vi "_DServerEventHandler.vi"(3 "error in":errorcluster, 4 "dserver evt.":T1, 5 "timeout":i32=250) -> (0 "error out":errorcluster, 1 "client request":T2={"Request Id"=0, "Source Id"=0, "Request Type"=enum."UNKNOWN_REQUEST", "Device Class Name"="unspecified_cmd_or_attr_name", "Device Name"="unspecified/device/name", "Cmd or Attr Name"="unspecified_cmd_or_attr_name", "Client Request Data"={"write attribute value"={"dimx"=0, "dimy"=0, "data"=[], "data_type"=enum."UNKNOWN_DATA_TYPE"}, "exec. command argin"={"num data"=[], "str data"=[]}}}, 2 "timeout":bool)   [LabVIEW 2014, in "tango.lvlib"]
uses:
  tango.lvlib
  Orphan/Typedefs/_DServerClientRequest.ctl
  Orphan/Typedefs/_DServerClientRequestType.ctl
  Orphan/Typedefs/_DServerClientRequestData.ctl
  Orphan/Typedefs/_GenericDataBuffer.ctl
  Orphan/Typedefs/_DataType.ctl
  Orphan/Typedefs/_DServerEvent.ctl
panel:
  in  "client request":T2={"Request Id"=0, "Source Id"=3, "Request Type"=enum."UNKNOWN_REQUEST", "Device Class Name"="unspecified_cmd_or_attr_name", "Device Name"="unspecified/device/name", "Cmd or Attr Name"="unspecified_cmd_or_attr_name", "Client Request Data"={"write attribute value"={"dimx"=0, "dimy"=0, "data"=[], "data_type"=enum."UNKNOWN_DATA_TYPE"}, "exec. command argin"={"num data"=[], "str data"=[]}}}
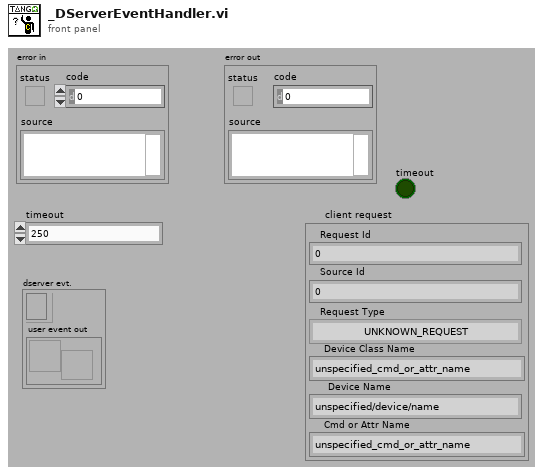
[diagram p1: front panel]
types:
  T1 = typedef "tango.lvlib/_DServerEvent.ctl" = cluster{"event registration refnum":refnum<event-registration>, "user event out":refnum<user-event>}
  T2 = typedef "tango.lvlib/_DServerClientRequest.ctl" = cluster{"Request Id":u32, "Source Id":u32, "Request Type":T3, "Device Class Name":string, "Device Name":string, "Cmd or Attr Name":string, "Client Request Data":T4}
  T3 = typedef "tango.lvlib/_DServerClientRequestType.ctl" = enum16{"EXEC_CMD", "READ_ATTR", "WRITE_ATTR", "UNKNOWN_REQUEST"}
  T4 = typedef "tango.lvlib/_DServerClientRequestData.ctl" = cluster{"write attribute value":T5, "exec. command argin":cluster{"num data":u8[], "str data":string[]}}
  T5 = typedef "tango.lvlib/_GenericDataBuffer.ctl" = cluster{"dimx":u32, "dimy":u32, "data":u8[], "data_type":T6}
  T6 = typedef "tango.lvlib/_DataType.ctl" = enum16{"STATE_SCA", "STATE_SPE", "STATE_IMG", "STRING_SCA", "STRING_SPE", "STRING_IMG", "BOOL_SCA", "BOOL_SPE", "BOOL_IMG", "UCHAR_SCA", "UCHAR_SPE", "UCHAR_IMG", "SHORT_SCA", "SHORT_SPE", "SHORT_IMG", "USHORT_SCA", "USHORT_SPE", "USHORT_IMG", "LONG_SCA", "LONG_SPE", "LONG_IMG", "ULONG_SCA", "ULONG_SPE", "ULONG_IMG", "LONG64_SCA", "LONG64_SPE", "LONG64_IMG", "ULONG64_SCA", "ULONG64_SPE", "ULONG64_IMG", "FLOAT_SCA", "FLOAT_SPE", "FLOAT_IMG", "DOUBLE_SCA", "DOUBLE_SPE", "DOUBLE_IMG", "SCA_ENCODED", "SPE_ENCODED", "IMG_ENCODED", "UNKNOWN_DATA_TYPE"}
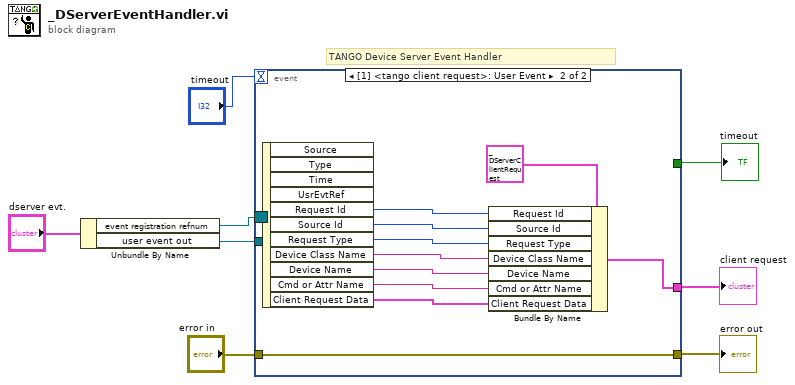
[diagram p0: block diagram]
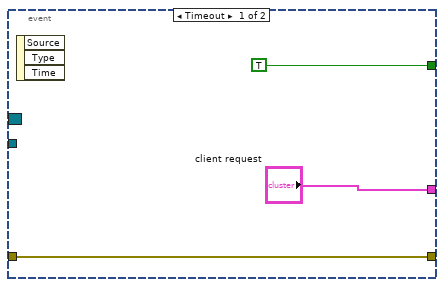
[diagram p2: hidden frame]
diagram:
  # "TANGO Device Server Event Handler"
  n1 = Unbundle By Name("dserver evt.") -> ("event registration refnum"=w2:refnum<event-registration>, "user event out"=w1:refnum<user-event>)
  n2 = event shown="[1] <tango client request>: User Event" {
    selector: w2 -> [_ _]
    dyn-events: _ -> [_ _]
    timeout: "timeout" -> [_ _]
    tunnel: "error in" -> [w11 w21]
    tunnel: [w11 w21] -> w7
    tunnel: [TRUE _] -> w5
    tunnel: ["client request" w13] -> w4
    tunnel: w1 -> [_ _]
    event Timeout {
      n3 = event-data() -> ()  [unwired: 1 in, 3 out]
    }
    event User Event {
      n4 = event-data() -> ("Request Id"=w19:u32, "Source Id"=w18:u32, "Request Type"=w17:T3, "Device Class Name"=w16:string, "Device Name"=w15:string, "Cmd or Attr Name"=w14:string, "Client Request Data"=w12:T4)  [unwired: 1 in, 4 out]
      n5 = Bundle By Name(cluster=T2 {"Request Id"=0, "Source Id"=0, "Request Type"=enum."UNKNOWN_REQUEST", "Device Class Name"="unspecified_class_name", "Device Name"="unspecified/device/name", "Cmd or Attr Name"="unspecified_cmd_or_attr_name", "Client Request Data"={"write attribute value"={"dimx"=0, "dimy"=0, "data"=[], "data_type"=enum."UNKNOWN_DATA_TYPE"}, "exec. command argin"={"num data"=[], "str data"=[]}}} ("Tango Client Request"), "Request Id"=w19, "Source Id"=w18, "Request Type"=w17, "Device Class Name"=w16, "Device Name"=w15, "Cmd or Attr Name"=w14, "Client Request Data"=w12) -> (w13:T2)
    }
  }
  "error out" <- w7
  "timeout" <- w5
  "client request" <- w4
